vi "save_vi.vi"(8 "error in (no error)":errorcluster, 10 "Path to Saved File":path, 11 "VI in":refnum<vi>) -> (0 "error out":errorcluster)   [LabVIEW 2020]
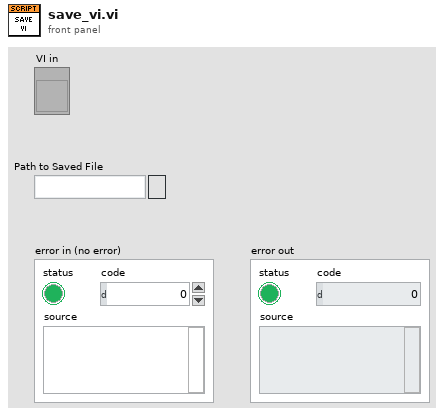
[diagram p1: front panel]
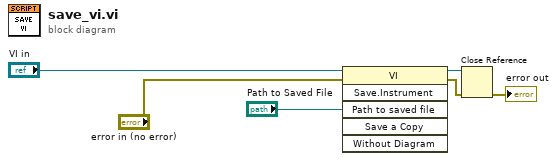
[diagram p0: block diagram]
diagram:
  n1 = invoke class="VI" method="Save.Instrument"(reference="VI in", error in="error in (no error)", "Path to saved file"="Path to Saved File") -> (reference out=w3:refnum<vi>, error out=w4:errorcluster)  [unwired: 3 in, 4 out]
  n2 = Close Reference(reference=w3, error in (no error)=w4) -> (error out=→"error out":errorcluster)
